vi "Configure Datalogger.vi"(8 "error in (no error)":errorcluster, 10 "Base File Path":path, 11 "Datalogger object in":refnum<class "Datalogger.lvclass">) -> (0 "error out":errorcluster, 3 "Datalogger object out":refnum<class "Datalogger.lvclass">)   [LabVIEW 2018, in "Datalogger.lvlib" / "Datalogger.lvclass"]
doc: "This VI sets the Base File Path for logging data to disk and then attempts to create/open a log file (Open Log File.vi). This will Open/Create a comma separated value(CSV) file"
uses:
  Datalogger.lvclass
  Datalogger.lvclass/Datalogger.ctl
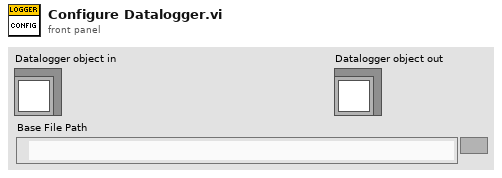
[diagram p1: front panel]
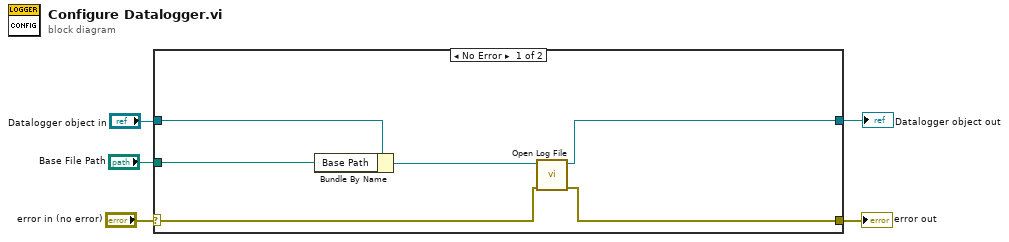
[diagram p0: block diagram]
diagram:
  n1 = case shown="No Error" "error in (no error)" {
    selector: "error in (no error)" -> [w7 w13]
    tunnel: [w6 w13] -> w4
    tunnel: "Datalogger object in" -> [w11 w12]
    tunnel: "Base File Path" -> [w10 _]
    tunnel: [w8 w12] -> w2
    frame No Error {
      n2 = Bundle By Name(cluster=w11, "Base Path"=w10) -> (w9:refnum<class "Datalogger.lvclass">)
      n3 = call "Open Log File.vi"("error in (no error)"=w7, "Datalogger Object In"=w9) -> ("error out"=w6:errorcluster, "Datalogger Object Out"=w8:refnum<class "Datalogger.lvclass">)  [unwired: 8 in]
    }
    frame Error {
    }
  }
  "error out" <- w4
  "Datalogger object out" <- w2
